vi "Network DAQ Control Event.vi"(0 "Control":T1, 2 "Mode (Set)":T2=enum."Set", 5 "Flattened Data":string, 11 "error in":errorcluster) -> (4 "Network DAQ Control Event Data":refnum<user-event>, 15 "error out":errorcluster)   [LabVIEW 2019]
uses:
  Type Defs and Controls/Event Mode Control.ctl
  Type Defs and Controls/Network DAQ Control Mode.ctl
  Type Defs and Controls/Network DAQ Control Event.ctl
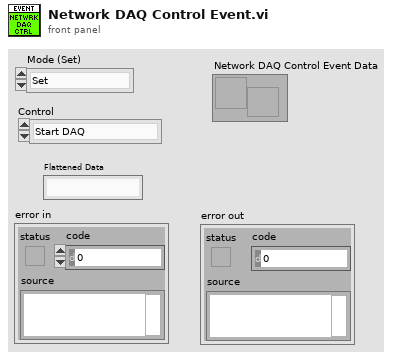
[diagram p1: front panel]
types:
  T1 = typedef "Network DAQ Control Mode.ctl" = enum16{"Start DAQ", "Stop DAQ"}
  T2 = typedef "Event Mode Control.ctl" = enum16{"Init", "Get", "Set", "Destroy"}
  T3 = typedef "Network DAQ Control Event.ctl" = cluster{"Data Type":T1, "Flattened Data":string}
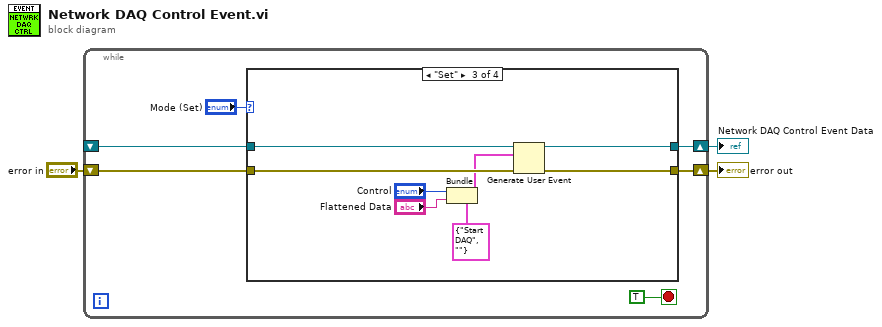
[diagram p0: block diagram]
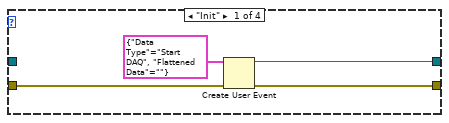
[diagram p2: hidden frame]
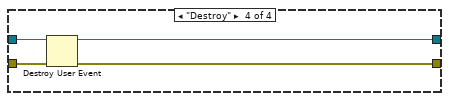
[diagram p4: hidden frame]
diagram:
  n1 = while {
    shift-right: [w7] -> w2
    shift-left: "error in" -> [w8]
    shift-right: [w5] -> w1
    shift-left: _ -> [w4]
    stop <- TRUE stop-if-true
    n2 = case shown="\"Set\"" "Mode (Set)" {
      tunnel: w8 -> [w13 w15 w23 w26]
      tunnel: [w12 w15 w22 w25] -> w7
      tunnel: [w10 w14 w17 w24] -> w5
      tunnel: w4 -> [_ w14 w18 w24]
      frame "Init" {
        n3 = Create User Event(user event datatype=T3 {"Data Type"=enum."Start DAQ", "Flattened Data"=""} ("CAN Control Event Data"), error in=w13) -> (user event=w10:refnum<user-event>, error out=w12:errorcluster)
      }
      frame "Get", Default {
      }
      frame "Set" {
        n4 = Bundle(cluster=T3 {"Data Type"=enum."Start DAQ", "Flattened Data"=""} ("CAN Control Event Data"), "Data Type"="Control", "Flattened Data"="Flattened Data") -> (w16:T3)
        n5 = Generate User Event(user event=w18, event data cluster=w16, error in=w23) -> (user event out=w17:refnum<user-event>, error out=w22:errorcluster)  [unwired: 1 in]
      }
      frame "Destroy" {
        n6 = Destroy User Event(user event=w24, error in=w26) -> (error out=w25:errorcluster)
      }
    }
  }
  "error out" <- w2
  "Network DAQ Control Event Data" <- w1
